vi "TaskMonitor.vi"() -> ()   [LabVIEW 2020]
panel:
  in  "ClearData":bool
  in  "TabMain":enum32{"Monitor", "Settings"}(tab)
  in  "Mem.UpdateTime":dbl=1.0 caption="UpdateTime" format="%0.3f sec"
  out "MemoryUsage":cluster{dbl, dbl}[](graph) caption="Memory Usage"
  out "CPU Load, %":cluster{dbl, dbl}[](graph)
  out "Mem.Instant":dbl caption="Instant" format="%0.0f  K"
  out "Mem.Max":dbl caption="Max" format="%0.0f  K"
  out "Mem.Min":dbl caption="Min" format="%0.0f  K"
  out "CPU.Load.Instant":dbl caption="Instant" format="%0.1f %"
  out "CPU.Load.Max":dbl caption="Max" format="%0.1f %"
  out "CPU.Load.Min":dbl caption="Min" format="%0.1f %"
  in  "ProcessList":i32(listbox)=-1
  in  "CPU.UpdateTime":dbl=1.0 caption="UpdateTime" format="%0.3f sec"
  out "error out":errorcluster
  in  "error in (no error)":errorcluster
  in  "Empty":bool
  in  "stop":bool
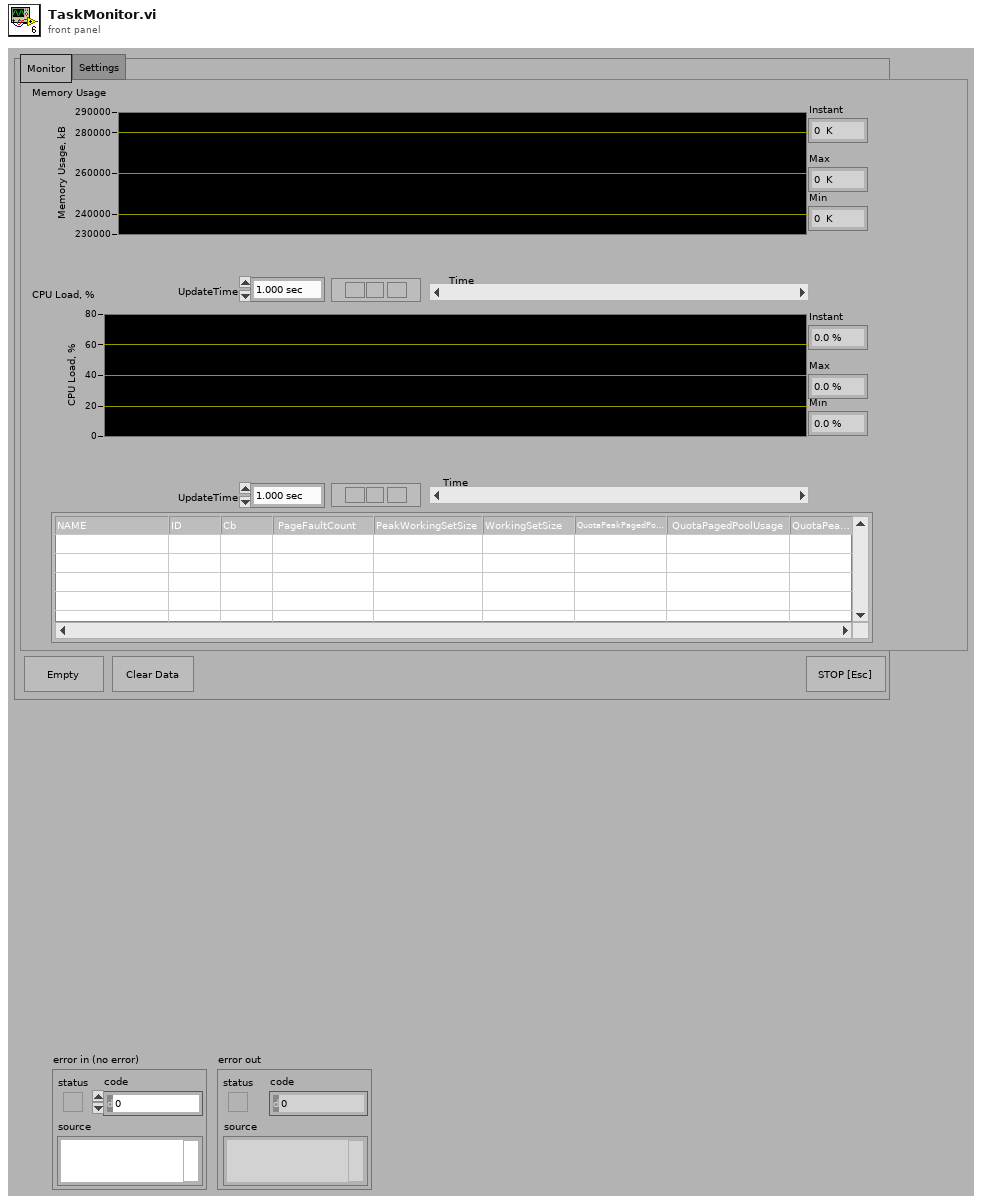
[diagram p1: front panel]
types:
  T1 = typedef "Labels&Control References.ctl" = cluster{"Refs":refnum<vi>[], "Labels":string[], "VI Ref":refnum<vi>}
  T2 = typedef "TaskMon_SynchronizationRef.ctl" = cluster{"STOP":refnum<notifier>, "PID":refnum<notifier>, "Process":refnum<notifier>}
  T3 = enum32{"invalid app kind", "Development System", "Run Time System", "Student Edition", "Embedded LabVIEW", "Evaluation", "Custom"}
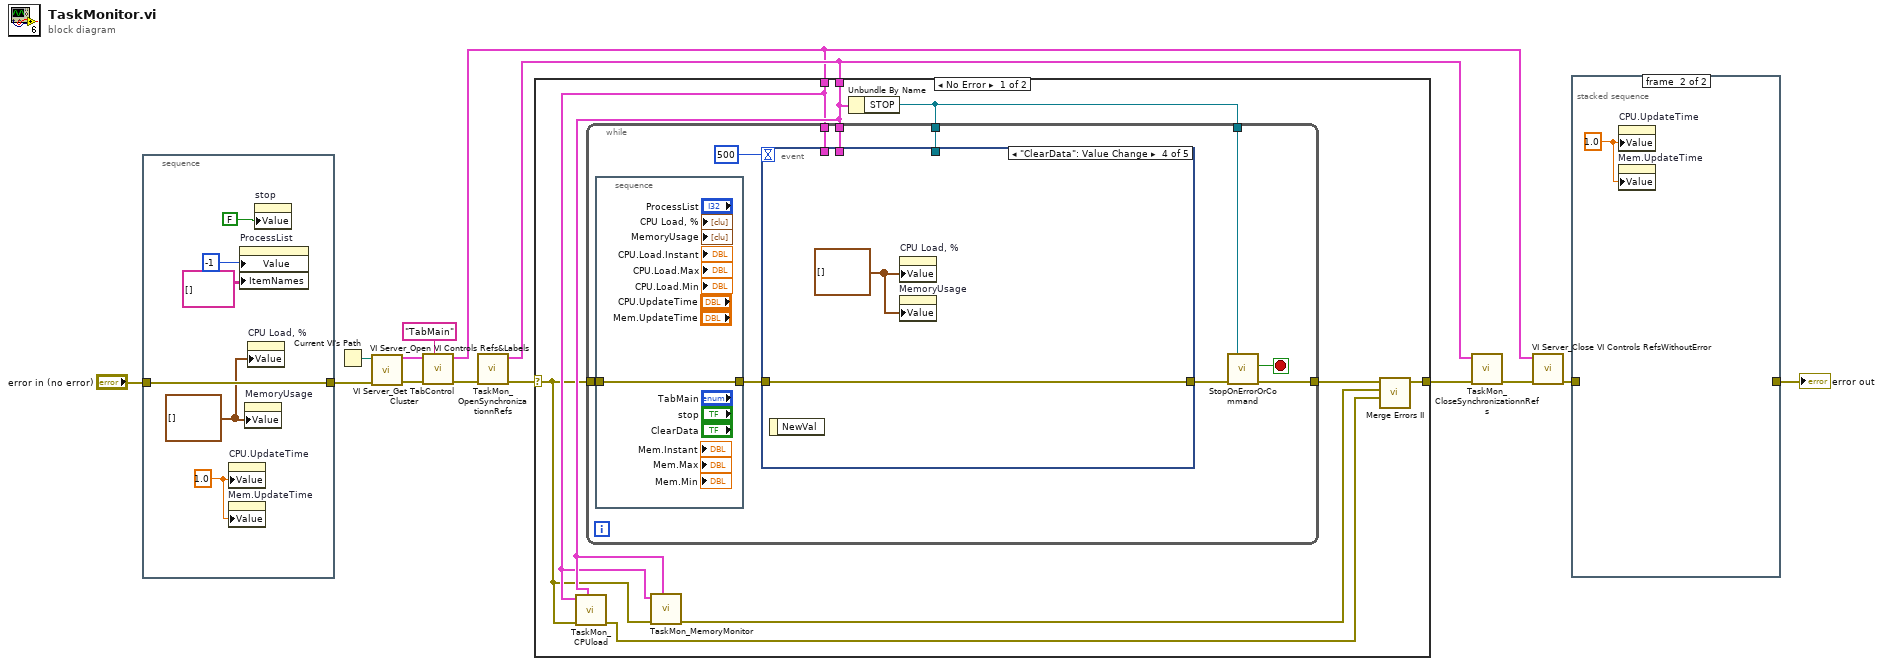
[diagram p0: block diagram]
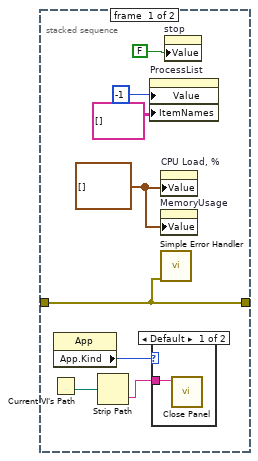
[diagram p2: hidden frame]
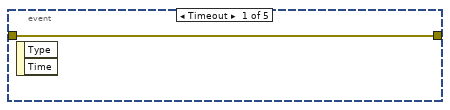
[diagram p4: hidden frame]
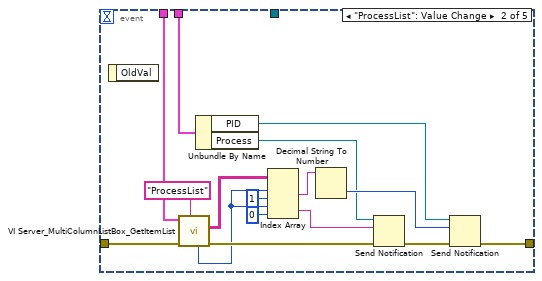
[diagram p5: hidden frame]
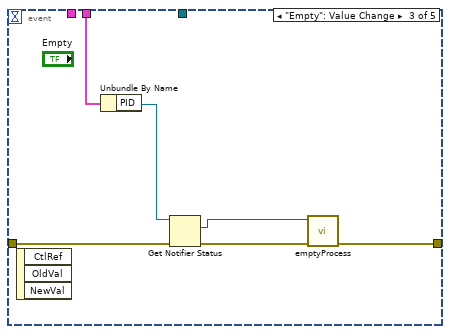
[diagram p6: hidden frame]
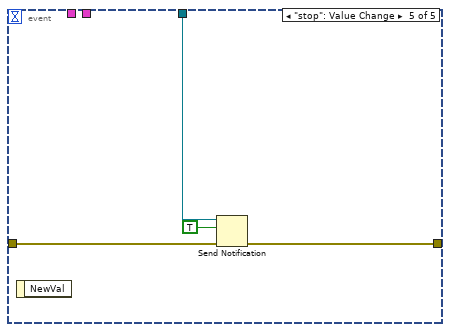
[diagram p7: hidden frame]
diagram:
  n1 = stacked-sequence {
    tunnel: "error in (no error)" -> [w19]
    tunnel: [w19] -> w13
    frame #0 {
      w15 = 1.0 ("CPU.UpdateTime")
      w16 = cluster{dbl, dbl}[] [] ("CPU Load, %")
      n2 = property on="CPU.UpdateTime" class="DigNum (strict)"("Value"=w15) -> ()  [unwired: 2 in, 2 out]
      n3 = property on="Mem.UpdateTime" class="DigNum (strict)"("Value"=w15) -> ()  [unwired: 2 in, 2 out]
      n4 = property on="ProcessList" class="MCListbox (strict)"("Value"=-1 ("ProcessList"), "ItemNames"=string[][] [] ("Item Names")) -> ()  [unwired: 2 in, 2 out]
      n5 = property on="MemoryUsage" class="XYGraph (strict)"("Value"=w16) -> ()  [unwired: 2 in, 2 out]
      n6 = property on="CPU Load, %" class="XYGraph (strict)"("Value"=w16) -> ()  [unwired: 2 in, 2 out]
      n7 = property on="stop" class="Bool (strict)"("Value"=FALSE ("stop")) -> ()  [unwired: 2 in, 2 out]
    }
  }
  n8 = Current VI's Path() -> (path=w12:path)
  n9 = call "VI Server_Open VI Controls Refs&Labels.vi"("error in (no error)"=w13, "vi path"=w12) -> ("error out"=w11:errorcluster, "Labels&Refs"=w10:T1)  [unwired: 8 in]
  n10 = call "VI Server_Get TabControl Cluster.vi"("TabControl Label"="TabMain", "error in"=w11, "VI Server Cluster.IN"=w10) -> ("error out"=w8:errorcluster, "VI Server Cluster.OUT"=w4:T1)  [unwired: 7 in]
  n11 = call "TaskMon_OpenSynchronizationnRefs.vi"("error in (no error)"=w8) -> ("error out"=w3:errorcluster, "SynchronizationRefs"=w5:T2)  [unwired: 9 in]
  n12 = case shown="No Error" w3 {
    selector: w3 -> [w21 w69]
    tunnel: [w27 w69] -> w6
    tunnel: w5 -> [w24 _]
    tunnel: w4 -> [w23 _]
    frame No Error {
      n13 = call "TaskMon_CPUload.vi"("SynchronizationRefs"=w24, "error in (no error)"=w21, "VI Server Cluster"=w23) -> ("error out"=w25:errorcluster)  [unwired: 7 in, 1 out]
      n14 = call "TaskMon_MemoryMonitor.vi"("SynchronizationRefs"=w24, "error in (no error)"=w21, "VI Server Cluster"=w23) -> ("error out"=w22:errorcluster)  [unwired: 8 in]
      n15 = Unbundle By Name(w24) -> ("STOP"=w28:refnum<notifier>)
      n16 = while {
        tunnel: w21 -> [w30]
        tunnel: [w34] -> w26
        tunnel: w23 -> [w37]
        tunnel: w24 -> [w36]
        tunnel: w28 -> [w32]
        tunnel: w28 -> [w31]
        stop <- w33 stop-if-true
        n17 = stacked-sequence {
          tunnel: w30 -> [w39]
          tunnel: [w39] -> w29
          frame #0 {
          }
        }
        n18 = event shown="[3] \"ClearData\": Value Change" {
          selector: _ -> [_ _ _ _ _]
          dyn-events: _ -> [_ _ _ _ _]
          timeout: 500 -> [_ _ _ _ _]
          tunnel: w29 -> [w40 w56 w59 w63 w67]
          tunnel: [w40 w41 w57 w63 w68] -> w35
          tunnel: w37 -> [_ w55 _ _ _]
          tunnel: w36 -> [_ w51 w62 _ _]
          tunnel: w31 -> [_ _ _ _ w66]
          event Timeout {
            n19 = event-data() -> ()  [unwired: 1 in, 2 out]
          }
          event "ProcessList": Value Change {
            n20 = event-data() -> ()  [unwired: 1 in, 1 out]
            n21 = call "VI Server_MultiColumnListBox_GetItemList.vi"("Label"="ProcessList", "error in"=w56, "Data Cluster"=w55) -> ("error out"=w48:errorcluster, "ItemNames"=w53:string[][], "Value"=w44:i32)  [unwired: 3 in, 3 out]
            n22 = Unbundle By Name(w51) -> ("PID"=w50:refnum<notifier>, "Process"=w46:refnum<notifier>)
            n23 = Index Array(array=w53, index (row) #1=w44, index (col) #1=1 ("disabled index (col)"), index (row) #2=w44, index (col) #2=0 ("disabled index (col)")) -> (element #1=w45:string, element #2=w42:string)
            n24 = Decimal String To Number(string=w45) -> (number=w49:i32)  [unwired: 2 in, 1 out]
            n25 = Send Notification(notification=w42, notifier=w46, error in (no error)=w48) -> (error out=w47:errorcluster)  [unwired: 1 out]
            n26 = Send Notification(notification=w49, notifier=w50, error in (no error)=w47) -> (error out=w41:errorcluster)  [unwired: 1 out]
          }
          event "Empty": Value Change {
            n27 = event-data() -> ()  [unwired: 1 in, 3 out]
            n28 = Unbundle By Name(w62) -> ("PID"=w61:refnum<notifier>)
            n29 = Get Notifier Status(notifier=w61, error in (no error)=w59) -> (current notification=w60:i32, error out=w58:errorcluster)  [unwired: 3 out]
            n30 = call "emptyProcess.vi"("error in (no error)"=w58, "ID"=w60) -> ("error out"=w57:errorcluster)  [unwired: 9 out]
          }
          event "ClearData": Value Change {
            w64 = cluster{dbl, dbl}[] [] ("CPU Load, %")
            n31 = event-data() -> ()  [unwired: 1 in, 1 out]
            n32 = property on="CPU Load, %" class="XYGraph (strict)"("Value"=w64) -> ()  [unwired: 2 in, 2 out]
            n33 = property on="MemoryUsage" class="XYGraph (strict)"("Value"=w64) -> ()  [unwired: 2 in, 2 out]
          }
          event "stop": Value Change {
            n34 = event-data() -> ()  [unwired: 1 in, 1 out]
            n35 = Send Notification(notification=TRUE, notifier=w66, error in (no error)=w67) -> (error out=w68:errorcluster)  [unwired: 1 out]
          }
        }
        n36 = call "StopOnErrorOrCommand.vi"("STOP"=w32, "error in (no error)"=w35) -> ("error out"=w34:errorcluster, "STOP"=w33:bool)  [unwired: 8 in]
      }
      n37 = call "Merge Errors II.vi"("error in 3 (no error)"=w25, "error in 2 (no error)"=w22, "error in 1 (no error)"=w26) -> ("error out.DUP"=w27:errorcluster)  [unwired: 3 in, 1 out]
    }
    frame Error {
    }
  }
  n38 = call "TaskMon_CloseSynchronizationnRefs.vi"("error in (no error)"=w6, "SynchronizationRefs"=w5) -> ("error out"=w7:errorcluster)  [unwired: 9 in]
  n39 = call "VI Server_Close VI Controls RefsWithoutError.vi"("error in (no error)"=w7, "Cluster"=w4) -> ("error out"=w2:errorcluster)  [unwired: 9 in]
  n40 = stacked-sequence {
    tunnel: w2 -> [w71 _]
    tunnel: [w71 _] -> w1
    frame #0 {
      w70 = cluster{dbl, dbl}[] [] ("CPU Load, %")
      n41 = Current VI's Path() -> (path=w72:path)
      n42 = property class="App"() -> ("App.Kind"=w73:T3)  [unwired: 2 in, 2 out]
      n43 = Strip Path(path=w72) -> (name=w74:string)  [unwired: 1 out]
      n44 = property on="ProcessList" class="MCListbox (strict)"("Value"=-1 ("ProcessList"), "ItemNames"=string[][] [] ("Item Names")) -> ()  [unwired: 2 in, 2 out]
      n45 = case shown="Default" w73 {
        tunnel: w74 -> [w78 _]
        frame Default {
          n46 = call <vilib>:"Close Panel.vi"("VI name"=w78) -> ()  [unwired: 1 in, 10 out]
        }
        frame "Development System" {
        }
      }
      n47 = property on="CPU Load, %" class="XYGraph (strict)"("Value"=w70) -> ()  [unwired: 2 in, 2 out]
      n48 = property on="MemoryUsage" class="XYGraph (strict)"("Value"=w70) -> ()  [unwired: 2 in, 2 out]
      n49 = call <vilib>:"Simple Error Handler.vi"("error in (no error)"=w71) -> ()  [unwired: 4 in, 5 out]
      n50 = property on="stop" class="Bool (strict)"("Value"=FALSE ("stop")) -> ()  [unwired: 2 in, 2 out]
    }
    frame #1 {
      w79 = 1.0 ("CPU.UpdateTime")
      n51 = property on="CPU.UpdateTime" class="DigNum (strict)"("Value"=w79) -> ()  [unwired: 2 in, 2 out]
      n52 = property on="Mem.UpdateTime" class="DigNum (strict)"("Value"=w79) -> ()  [unwired: 2 in, 2 out]
    }
  }
  "error out" <- w1
